vi "Shift.vi"(1 "Shift by":i32=1, 2 "A":T1={"Array Num"=[1, 2, 3], "Decimal Index"=0, "stop"=FALSE}) -> (0 "Shifted A":T1={"Array Num"=[1, 2, 3], "Decimal Index"=0, "stop"=FALSE})   [LabVIEW 2025]
uses:
  Number.ctl
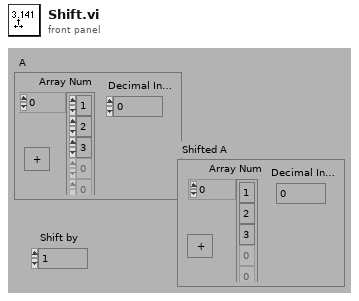
[diagram p1: front panel]
types:
  T1 = typedef "Number.ctl" = cluster{"Array Num":i8[], "Decimal Index":i32, "stop":bool}
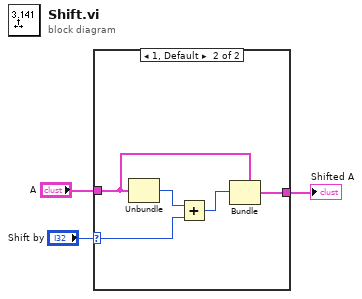
[diagram p0: block diagram]
diagram:
  n1 = case shown="1, Default" "Shift by" {
    selector: "Shift by" -> [_ w5]
    tunnel: "A" -> [w4 w8]
    tunnel: [w4 w6] -> w2
    frame 0 {
    }
    frame 1, Default {
      n2 = Unbundle(w8) -> ("Decimal Index"=w9:i32)  [unwired: 2 out]
      n3 = Add(x=w9, y=w5) -> (x+y=w7:i32)
      n4 = Bundle(cluster=w8, "Decimal Index"=w7) -> (w6:T1)  [unwired: 2 in]
    }
  }
  "Shifted A" <- w2
